vi "Horst-Test.vi"() -> ()   [LabVIEW 2017]
uses:
  <vilib>/Utility/error.llb/Error Cluster From Error Code.vi
  <vilib>/rvi/errors/niLvFpgaAdjustHostInterfaceError.vi
  <vilib>/FPGAPlugInAG/cRIO-9035/niLvFpga_Close_cRIO-9035.vi
  <vilib>/rvi/interface/nirviMethod/nirviMethod.xnode
  FPGA Bitfiles/HAGAR-VECD_FPGATarget_FPGA-ProgrammECD_WS++LmW9gGg.lvbitx
  FPGA-Programm_ECD.vi
  <vilib>/rvi/interface/nirviReadWriteControl/nirviReadWriteControl.xnode
  <vilib>/rvi/interface/nirviCloseFPGA/nirviCloseFPGA.xnode
  <vilib>/rvi/errors/niLvFpgaMergeErrorWithErrorCode.vi
  <vilib>/FPGAPlugInAG/cRIO-9035/niLvFpga_ReadFifo_cRIO-9035.vi
  <vilib>/FPGAPlugInAG/cRIO-9035/niLvFpga_WriteFifo_cRIO-9035.vi
  NiFpgaLv.dll
panel:
  in  "Index":i32
  in  "Array":string[](array[string])
  out "stop":errorcluster caption="Fehler (Ausgang)"
  out "empfangen":string
  out "Fehler (Ausgang)":errorcluster
  in  "senden":bool
  in  "Stopp":bool
  out "FPGA-Start":errorcluster caption="error out"
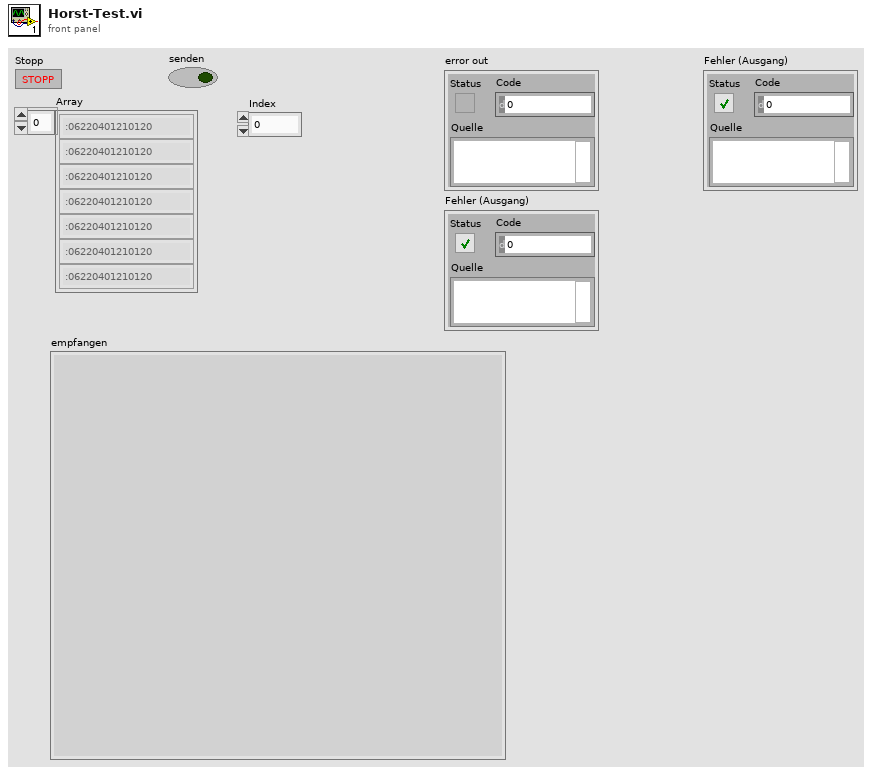
[diagram p1: front panel]
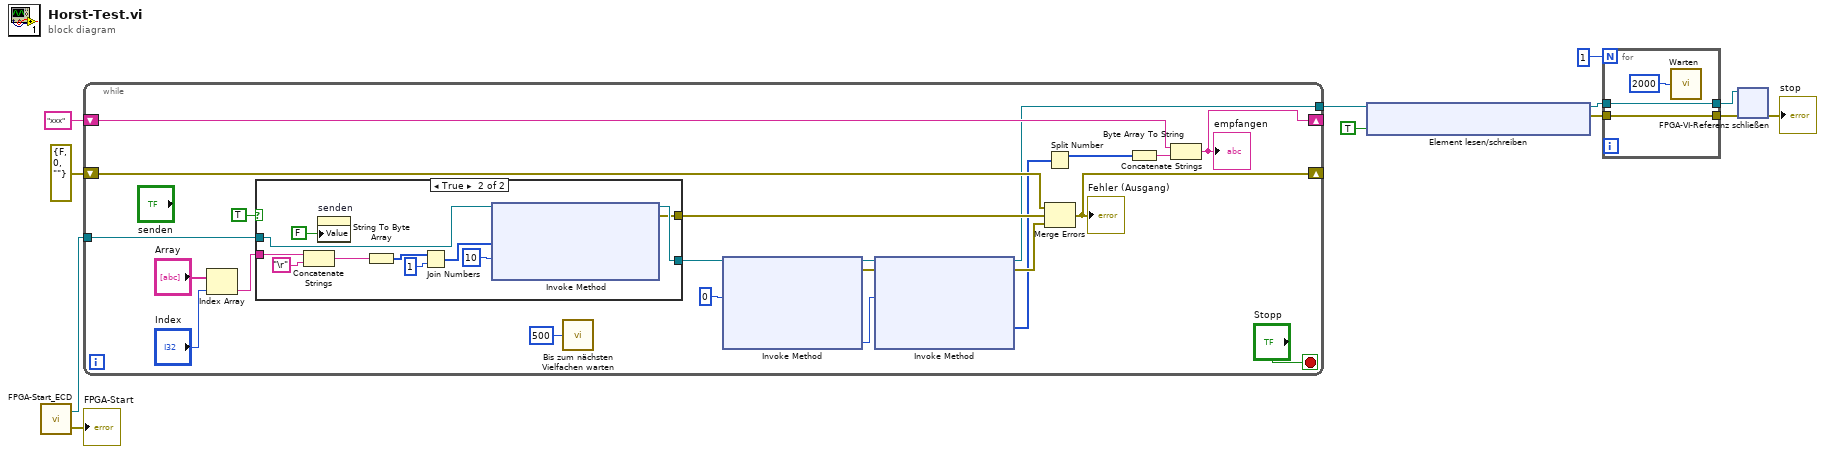
[diagram p0: block diagram]
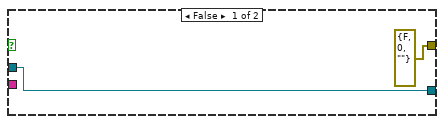
[diagram p2: hidden frame]
diagram:
  n1 = call "FPGA-Start_ECD.vi"() -> ("error out"=→"FPGA-Start":errorcluster, "FPGA-VI-Referenz (Ausgang)"=w12:refnum<k20>)  [unwired: 2 in]
  n2 = while {
    tunnel: w12 -> [w34]
    shift-right: [w25] -> _
    shift-left: errorcluster {"status"=FALSE, "code"=0, "source"=""} ("error IO") -> [w33]
    shift-right: [w19] -> _
    shift-left: "xxx" -> [w22]
    tunnel: [w20] -> w8
    stop <- "Stopp" stop-if-true
    n3 = Index Array(array="Array", index="Index") -> (element=w16:string)
    n4 = case shown="True" TRUE {
      tunnel: w34 -> [w36 w41]
      tunnel: [w36 w40] -> w31
      tunnel: w16 -> [_ w39]
      tunnel: [errorcluster {"status"=FALSE, "code"=0, "source"=""} ("Fehler (Ausgang)") w38] -> w32
      frame False {
      }
      frame True {
        n5 = Concatenate Strings(w39, "\r") -> (w42:string)
        n6 = property on="senden" class="Bool. (strikt)"("Value"=FALSE ("senden")) -> ()  [unwired: 2 in, 2 out]
        n7 = String To Byte Array(string=w42) -> (unsigned byte array=w47:u8[])
        n8 = Join Numbers(hi=w47, lo=u8 1) -> ((hi.lo)=w45:u16[])
        n9 = xnode "Invoke Method"("FPGA-VI-Referenz (Eingang)"=w41, "Daten"=w45, "Timeout (ms)"=10) -> ("FPGA-VI-Referenz (Ausgang)"=w40:refnum<k20>, "Fehler (Ausgang)"=w38:errorcluster)  [unwired: 1 in, 1 out]
      }
    }
    n10 = call "Bis zum nächsten Vielfachen warten"("Count(mSec)"=u32 500) -> ()  [unwired: 1 out]
    n11 = xnode "Invoke Method"("FPGA-VI-Referenz (Eingang)"=w31, "Anzahl der Elemente"=u32 0) -> ("FPGA-VI-Referenz (Ausgang)"=w30:refnum<k20>, "Fehler (Ausgang)"=w27:errorcluster, "Verbleibende Elemente"=w28:u32)  [unwired: 2 in, 1 out]
    n12 = xnode "Invoke Method"("FPGA-VI-Referenz (Eingang)"=w30, "Fehler (Eingang)"=w27, "Anzahl der Elemente"=w28) -> ("FPGA-VI-Referenz (Ausgang)"=w20:refnum<k20>, "Fehler (Ausgang)"=w26:errorcluster, "Daten"=w24:u16[])  [unwired: 1 in, 1 out]
    n13 = Split Number(x=w24) -> (hi(x)=w15:u8[])  [unwired: 1 out]
    n14 = Merge Errors(w33, w32, w26) -> (w25:errorcluster)
    "Fehler (Ausgang)" <- w25
    n15 = Byte Array To String(unsigned byte array=w15) -> (string=w23:string)
    n16 = Concatenate Strings(w22, w23) -> (w19:string)
    "empfangen" <- w19
  }
  n17 = xnode "Element lesen/schreiben"("FPGA-VI-Referenz (Eingang)"=w8, "global stop"=TRUE) -> ("FPGA-VI-Referenz (Ausgang)"=w6:refnum<k20>, "Fehler (Ausgang)"=w5:errorcluster)  [unwired: 1 in]
  n18 = for {
    N: 1 -> [_]
    tunnel: w6 -> [w49]
    tunnel: w5 -> [w48]
    tunnel: [w49] -> w4
    tunnel: [w48] -> w3
    n19 = call "Warten"("Count(mSec)"=u32 2000) -> ()  [unwired: 1 out]
  }
  n20 = xnode "FPGA-VI-Referenz schließen"("FPGA-VI-Referenz (Eingang)"=w4, "Fehler (Eingang)"=w3) -> ("Fehler (Ausgang)"=→"stop":errorcluster)
